vi "Not A Known Hosts Collection.vi"(1 "known hosts collection":T1) -> (0 "Not a Known Hosts Collection?":bool)   [LabVIEW 2013, in "libssh2.lvlib"]
doc: "Returns TRUE if <B>known host collection</B> is not a known host collection. Otherwise, this function returns FALSE."
uses:
  libssh2.lvlib
  Known Hosts Collection Refnum.ctl
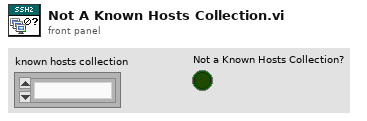
[diagram p1: front panel]
types:
  T1 = typedef "libssh2.lvlib/Known Hosts Collection Refnum.ctl" = refnum<k1>
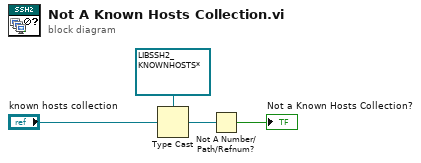
[diagram p0: block diagram]
diagram:
  n1 = Type Cast(type=refnum<data-value> refnum ("data value reference"), x="known hosts collection") -> (*(type *) &x=w2:refnum<data-value>)
  n2 = Not A Number/Path/Refnum?(number/path/refnum=w2) -> (NaN/Path/Refnum?=→"Not a Known Hosts Collection?":bool)
